vi "receive rig channels.vi"(8 "customViData in":T2, 10 "data":variant) -> (0 "customViData out":T2, 2 "updated plotControl":T1[](array[typedef]))   [LabVIEW 2018]
uses:
  customViData.ctl
  plotControl.ctl
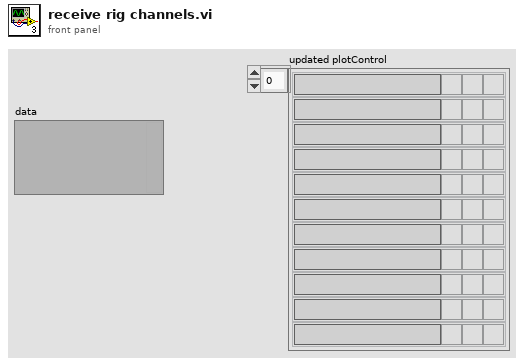
[diagram p1: front panel]
types:
  T1 = typedef "plotControl.ctl" = cluster{"channel":string, "X":bool, "Y":bool, "Y2":bool}
  T2 = typedef "customViData.ctl" = cluster{"rigChannels":string[], "rigUnits":string[], "logging":bool, "plot":cluster{"X":u16[], "Y":u16[], "Y2":u16[]}, "updatePlot":bool, "chartRef":refnum<vi>, "livePlot":bool, "history":dbl[][], "channelCount":i32, "trendIndex":i32}
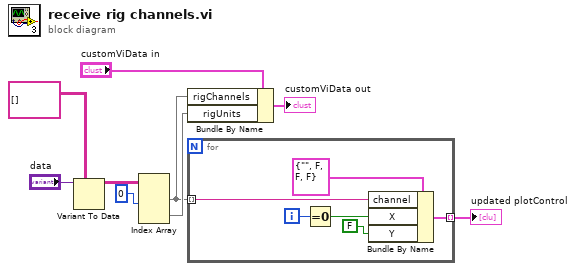
[diagram p0: block diagram]
diagram:
  n1 = Variant To Data(type=string[][] [], Variant="data") -> (data=w7:string[][])  [unwired: 1 in, 1 out]
  n2 = Index Array(array=w7, index (col) #1=0 ("index (row)")) -> (element #1=w2:string[], element #2=w8:string[])  [unwired: 3 in]
  n3 = Bundle By Name(cluster="customViData in", "rigChannels"=w2, "rigUnits"=w8) -> (→"customViData out":T2)
  n4 = for {
    tunnel: w2 -> [w13] mode=indexing
    tunnel: [w14] -> w1 mode=indexing
    i -> [w11]
    n5 = Equal To 0?(x=w11) -> (x = 0?=w12:bool)
    n6 = Bundle By Name(cluster=T1 {"channel"="", "X"=FALSE, "Y"=FALSE, "Y2"=FALSE} ("Plot Control"), "channel"=w13, "X"=w12, "Y"=FALSE) -> (w14:T1)
  }
  "updated plotControl" <- w1
